vi "fgv_feedback_counter.vi"(9 "function":T1, 11 "data in":i32) -> (3 "data out":i32)   [LabVIEW 2021]
doc: "本VI是为《我和LabVIEW》一书编写的示例。\n关于本书的介绍请参考网页：\nhttp://ruanqizhen.spaces.live.com/blog/cns!5852D4F797C53FB6!4310.entry"
uses:
  fgv_function.ctl
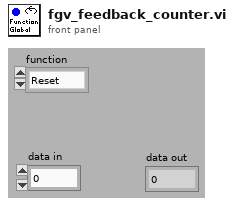
[diagram p1: front panel]
types:
  T1 = typedef "fgv_function.ctl" = enum16{"Reset", "Increase", "Decrease", "Read"}
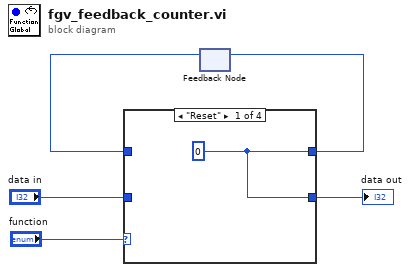
[diagram p0: block diagram]
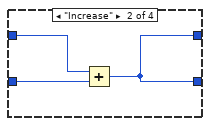
[diagram p2: hidden frame]
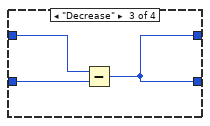
[diagram p3: hidden frame]
diagram:
  n1 = feedback #1() -> (w1:i32)  [unwired: 1 in]
  n2 = case shown="\"Reset\"" "function" {
    tunnel: [w6 w7 w10 w13] -> w3
    tunnel: w1 -> [_ w9 w12 w13]
    tunnel: "data in" -> [_ w8 w11 _]
    tunnel: [w6 w7 w10 w13] -> w2
    frame "Reset" {
      w6 = 0
    }
    frame "Increase" {
      n3 = Add(x=w9, y=w8) -> (x+y=w7:i32)
    }
    frame "Decrease" {
      n4 = Subtract(x=w12, y=w11) -> (x-y=w10:i32)
    }
    frame "Read" {
    }
  }
  "data out" <- w3
  n5 = feedback-in #1(w2) -> ()
